vi "StateDrivebase.vi"(0 "Master State In":T1(ring)) -> ()   [LabVIEW 2020]
doc: "This VI performs all of the calculations and decisions related to the swerve drive."
uses:
  GlobalDriverStationCommands.vi
  GlobalDriverStationData.vi
  GlobalPoseAndTargeting.vi
  GlobalDrivebase.vi
panel:
  in  "Max Strafing While Balancing":dbl=0.25
  in  "Speed Cap Decceleration Limit (/s)":dbl=20.0
  in  "PID Tuning Anti-Drift":T2={"Kp"=0.00045, "Ki"=0.0, "Kd"=0.0, "N-Diff"=3, "N-Int"=10, "Int Error Window"=90.0, "Max Ouput"=1.0, "Min Output"=-1.0, "Square Derivative"=FALSE, "N-Prop"=5} {"N-Prop" min=1; "Int Error Window" min=0.0; "N-Int" min=2; "N-Diff" min=2; "Kd" min=0.0; "Ki" min=0.0; "Kp" min=0.0}
  in  "Anti-Drift Deceleration Hysteresis (ms)":u32=1
  out "Anti-Drift Control":bool
  in  "Anti-Drift Strafe Deadband (ft/s)":dbl=3.0
  in  "Manually Disable Anti-Drift":bool
  in  "PID Tuning Heading Lock":T3={"Kp"=0.0045, "Ki"=0.01, "Kd"=0.0002, "N-Diff"=10, "N-Int"=10, "Int Error Window"=30.0, "Max Ouput"=1.0, "Min Output"=-1.0} {"Int Error Window" min=0.0; "N-Int" min=2; "N-Diff" min=2; "Kd" min=0.0; "Ki" min=0.0; "Kp" min=0.0}
  out "PID Plots":T4(graph)
  in  "Manual Fudge Factor Heading Lock (deg)":dbl=10.0
  in  "Plot PID":bool
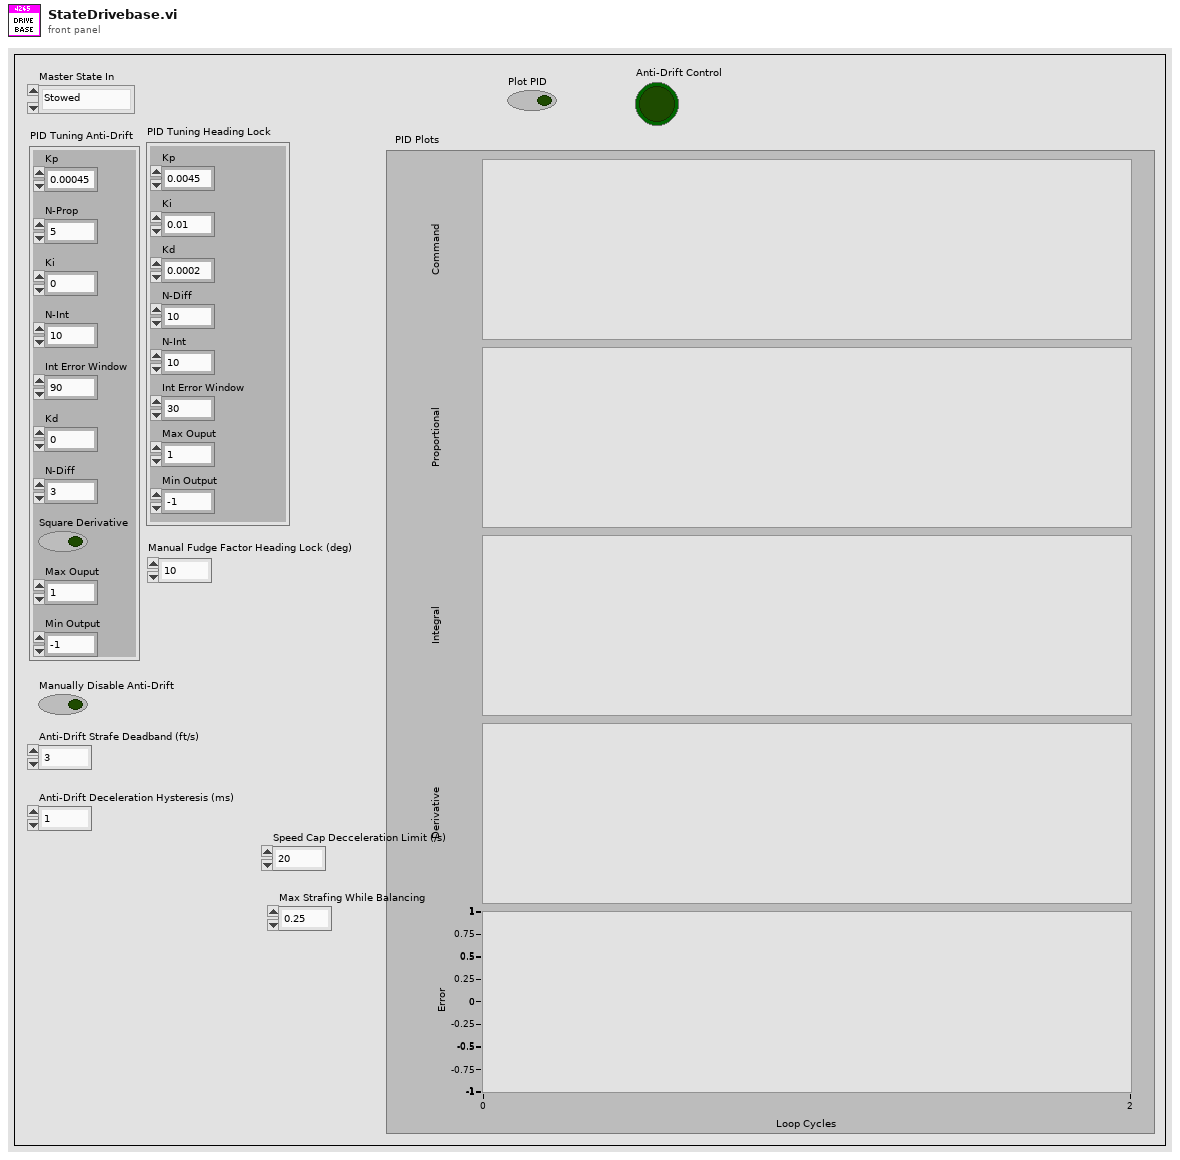
[diagram p1: front panel]
types:
  T1 = enum16{"Stowed", "Balancing", "Scoring", "Hoppering", "Ground", "Shelf"}
  T2 = cluster{"Kp":dbl, "Ki":dbl, "Kd":dbl, "N-Diff":i32, "N-Int":i32, "Int Error Window":dbl, "Max Ouput":dbl, "Min Output":dbl, "Square Derivative":bool, "N-Prop":i32}
  T3 = cluster{"Kp":dbl, "Ki":dbl, "Kd":dbl, "N-Diff":i32, "N-Int":i32, "Int Error Window":dbl, "Max Ouput":dbl, "Min Output":dbl}
  T4 = cluster{"Command":dbl, "Proportional":dbl, "Integral":dbl, "Derivative":dbl, "Goal":dbl}
  T5 = cluster{"Current Setpoints[0]":dbl, "Current Setpoints[1]":dbl, "Current Setpoints[2]":dbl, "Current Setpoints[3]":dbl, "Current Setpoints[4]":dbl, "Current Setpoints[5]":dbl, "Current Setpoints[6]":dbl, "Current Setpoints[7]":dbl, "Current Setpoints[8]":dbl}
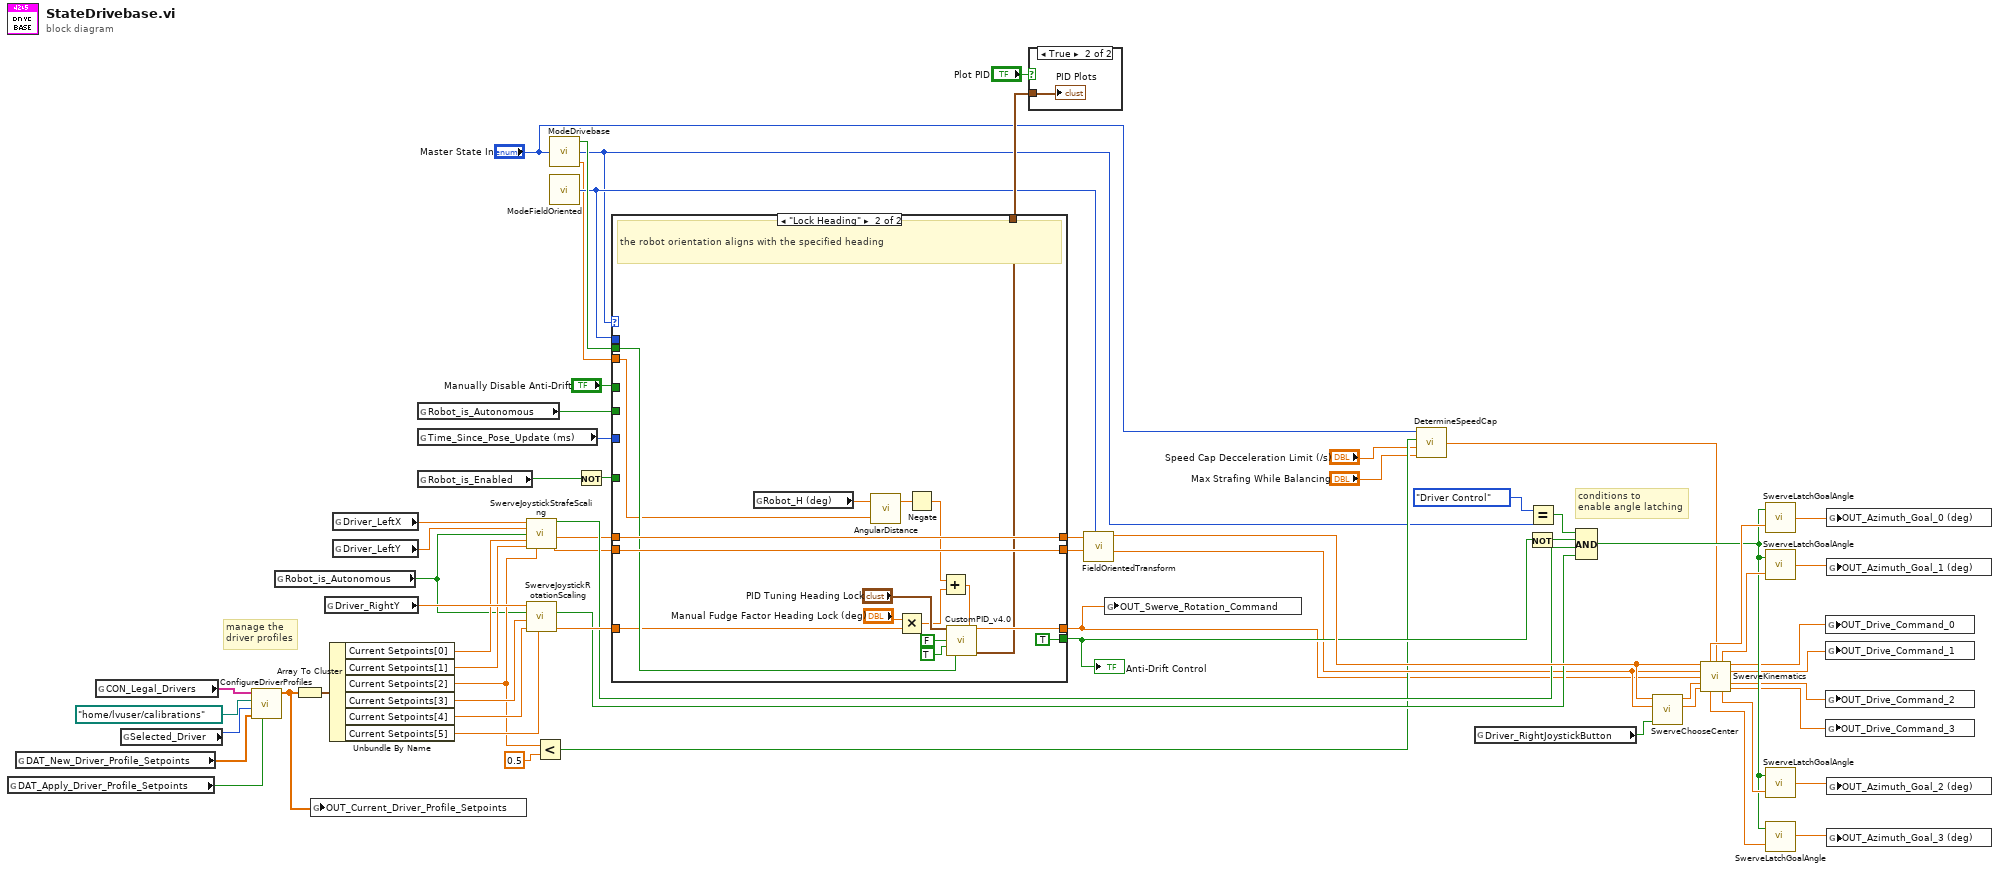
[diagram p0: block diagram]
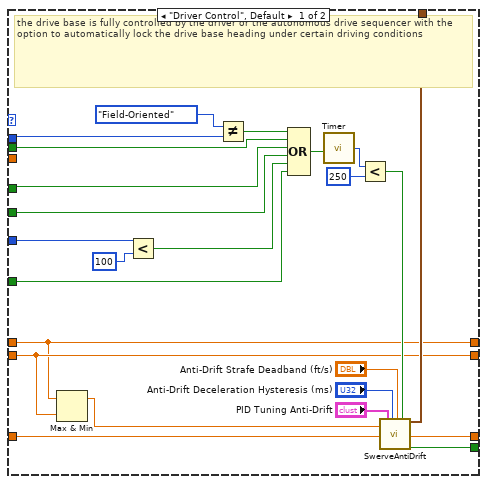
[diagram p3: hidden frame]
diagram:
  # "conditions to\nenable angle latching"
  # "manage the\ndriver profiles"
  n1 = global read "GlobalDrivebase.vi" "DAT_Apply_Driver_Profile_Setpoints"() -> (w20:bool)
  n2 = global read "GlobalDrivebase.vi" "DAT_New_Driver_Profile_Setpoints"() -> (w21:dbl[])
  n3 = global read "GlobalDrivebase.vi" "CON_Legal_Drivers"() -> (w19:string[])
  n4 = global read "GlobalDriverStationData.vi" "Selected_Driver"() -> (w31:i32)
  n5 = call "ConfigureDriverProfiles.vi"("Apply New Setpoint"=w20, "New Setpoints"=w21, "Selected Driver"=w31, "Setpoint Save Location"=path "/home/lvuser/calibrations", "Driver Profile Names"=w19) -> ("Current Setpoints"=w9:dbl[])  [unwired: 6 in]
  n6 = global read "GlobalDriverStationData.vi" "Robot_is_Autonomous"() -> (w27:bool)
  n7 = Array To Cluster(array=w9) -> (cluster=w30:T5)
  n8 = global write "GlobalDrivebase.vi" "OUT_Current_Driver_Profile_Setpoints"(w9) -> ()
  n9 = global read "GlobalDriverStationCommands.vi" "Driver_RightY"() -> (w49:dbl)
  n10 = Unbundle By Name(w30) -> ("Current Setpoints[0]"=w39:dbl, "Current Setpoints[1]"=w38:dbl, "Current Setpoints[2]"=w28:dbl, "Current Setpoints[3]"=w37:dbl, "Current Setpoints[4]"=w36:dbl, "Current Setpoints[5]"=w35:dbl)
  n11 = global read "GlobalDriverStationCommands.vi" "Driver_LeftX"() -> (w52:dbl)
  n12 = global read "GlobalDriverStationCommands.vi" "Driver_LeftY"() -> (w51:dbl)
  n13 = global read "GlobalDriverStationData.vi" "Robot_is_Autonomous"() -> (w57:bool)
  n14 = global read "GlobalPoseAndTargeting.vi" "Time_Since_Pose_Update (ms)"() -> (w58:u32)
  n15 = global read "GlobalDriverStationData.vi" "Robot_is_Enabled"() -> (w6:bool)
  n16 = call "SwerveJoystickStrafeScaling.vi"("Raw Joystick X"=w52, "Raw Joystick Y"=w51, "Auto Control"=w27, "Strafe Deadband"=w39, "Strafe Scaling"=w38, "Strafe Maximum"=w28) -> ("In Deadband"=w45:bool, "Scaled Joystick X"=w25:dbl, "Scaled Joystick Y"=w26:dbl)  [unwired: 7 in]
  n17 = call "SwerveJoystickRotationScaling.vi"("Rotation Maximum"=w35, "Rotation Scaling"=w36, "Rotation Deadband"=w37, "Auto Control"=w27, "Raw Joystick Rotation"=w49) -> ("Scaled Joystick Rotation"=w50:dbl, "In Deadband"=w46:bool)  [unwired: 4 in]
  n18 = Less?(x=w28, y=0.5) -> (x < y?=w22:bool)
  n19 = call "ModeDrivebase.vi"("Master State In"="Master State In") -> ("Drive Mode Change"=w55:bool, "Drive Mode"=w4:enum16{"Driver Control", "Lock Heading"}, "Locked Heading (deg)"=w7:dbl)
  n20 = call "ModeFieldOriented.vi"() -> ("Orientation Mode"=w41:enum16{"Robot-Oriented", "Field-Oriented"})  [unwired: 1 in]
  n21 = Not(x=w6) -> (.not. x?=w5:bool)
  n22 = case shown="\"Lock Heading\"" w4 {
    tunnel: [w68 w104] -> w40
    tunnel: [w67 w102] -> w64
    tunnel: w25 -> [w67 w102]
    tunnel: w26 -> [w68 w104]
    tunnel: w50 -> [w79 w90]
    tunnel: [w80 w101] -> w18
    tunnel: [w85 TRUE ("auto rot control")] -> w47
    tunnel: w41 -> [w86 _]
    tunnel: w57 -> [w83 _]
    tunnel: w55 -> [w77 w97]
    tunnel: w58 -> [w88 _]
    tunnel: [w82 w96] -> w56
    tunnel: "Manually Disable Anti-Drift" -> [w81 _]
    tunnel: w5 -> [w71 _]
    tunnel: w7 -> [_ w91]
    frame "Driver Control", Default {
      # "the drive base is fully controlled by the driver or the autonomous drive sequencer with the option to automatically lock the drive base heading under certain driving conditions"
      n23 = Max & Min(x=w67, y=w68) -> (max(x,y)=w66:dbl)  [unwired: 1 out]
      n24 = Less?(x=w88, y=u32 100) -> (x < y?=w84:bool)
      n25 = Not Equal?(x=enum16{"Robot-Oriented", "Field-Oriented"}."Field-Oriented", y=w86) -> (x != y?=w76:bool)
      n26 = Compound Arithmetic op=OR(w76, w77, w81, w83, w84, w71) -> (w74:bool)
      n27 = call "Timer.vi"("Reset Timer"=w74) -> ("Time (ms)"=w75:u32)
      n28 = Less?(x=w75, y=u32 250) -> (x < y?=w72:bool)
      n29 = call "SwerveAntiDrift.vi"("Max Driver Translation Joystick"=w66, "Driver Rotation Joystick"=w79, "PID Tuning Parameters"="PID Tuning Anti-Drift", "Deceleration Hysteresis (ms)"="Anti-Drift Deceleration Hysteresis (ms)", "Strafe Deadband (ft/s)"="Anti-Drift Strafe Deadband (ft/s)", "External Disables"=w72) -> ("Controller Summary"=w82:T4, "Joystick Rotation"=w80:dbl, "Anti-Drift"=w85:bool)  [unwired: 11 in]
    }
    frame "Lock Heading" {
      # "the robot orientation aligns with the specified heading"
      n30 = global read "GlobalPoseAndTargeting.vi" "Robot_H (deg)"() -> (w105:dbl)
      n31 = call "AngularDistance.vi"("Goal Angle (deg) [0,360]"=w91, "Current Angle (deg) [-Inf,+Inf]"=w105) -> ("Signed Angular Distance (deg) [-180,+180]"=w95:dbl)  [unwired: 1 out]
      n32 = Multiply(x="Manual Fudge Factor Heading Lock (deg)", y=w90) -> (x*y=w94:dbl)
      n33 = Negate(x=w95) -> (-x=w93:dbl)
      n34 = Add(x=w93, y=w94) -> (x+y=w92:dbl)
      n35 = call "CustomPID_v4.0.vi"("PID Tuning Parameters"="PID Tuning Heading Lock", "Custom Error Calculation"=w92, "Reset on Goal Change ?"=FALSE, "Use Custom Error Calculation ?"=TRUE, "Reinit"=w97) -> ("Command"=w101:dbl, "Controller Summary"=w96:T4)  [unwired: 7 in, 2 out]
    }
  }
  "Anti-Drift Control" <- w47
  n36 = case shown="True" "Plot PID" {
    tunnel: w56 -> [_ w106]
    frame False {
    }
    frame True {
      "PID Plots" <- w106
    }
  }
  n37 = call "FieldOrientedTransform.vi"("Orientation Mode"=w41, "Joystick Y"=w40, "Joystick X"=w64) -> ("Joystick Y'"=w42:dbl, "Joystick X'"=w48:dbl)  [unwired: 7 in]
  n38 = global write "GlobalDrivebase.vi" "OUT_Swerve_Rotation_Command"(w18) -> ()
  n39 = call "DetermineSpeedCap.vi"("Max Strafing While Balancing"="Max Strafing While Balancing", "Speed Cap Decceleration Limit (/s)"="Speed Cap Decceleration Limit (/s)", "Driver Profile Doesn't Want to Shift"=w22, "Master State"="Master State In") -> ("Speed Cap [0,1]"=w23:dbl)
  n40 = global read "GlobalDriverStationCommands.vi" "Driver_RightJoystickButton"() -> (w54:bool)
  n41 = Not(x=w47) -> (.not. x?=w44:bool)
  n42 = Equal?(x=enum16{"Driver Control", "Lock Heading"}."Driver Control" ("Drive Mode"), y=w4) -> (x = y?=w43:bool)
  n43 = Compound Arithmetic op=AND(w43, w44, w45, w46) -> (w24:bool)
  n44 = call "SwerveChooseCenter.vi"("Defensive Driving Trigger"=w54, "Joystick Y"=w42, "Joystick X"=w48) -> ("Cy (in)"=w33:dbl, "Cx (in)"=w34:dbl)  [unwired: 5 in]
  n45 = call "SwerveKinematics.vi"("Joystick X"=w48, "Saturation Velocity (ul)"=w23, "Joystick Y"=w42, "Joystick Rotation"=w18, "Cx (in)"=w34, "Cy (in)"=w33) -> ("Module 0 Angle (deg)"=w63:dbl, "Module 1 Angle (deg)"=w62:dbl, "Module 0 Velocity Command (ul)"=w13:dbl, "Module 1 Velocity Command (ul)"=w12:dbl, "Module 2 Velocity Command (ul)"=w11:dbl, "Module 3 Angle (deg)"=w59:dbl, "Module 2 Angle (deg)"=w60:dbl, "Module 3 Velocity Command (ul)"=w10:dbl)  [unwired: 2 in]
  n46 = call "SwerveLatchGoalAngle.vi"("Raw Goal Angle"=w63, "In Deadband"=w24) -> ("Latched Goal Angle"=w17:dbl)
  n47 = call "SwerveLatchGoalAngle.vi"("Raw Goal Angle"=w62, "In Deadband"=w24) -> ("Latched Goal Angle"=w16:dbl)
  n48 = call "SwerveLatchGoalAngle.vi"("Raw Goal Angle"=w60, "In Deadband"=w24) -> ("Latched Goal Angle"=w15:dbl)
  n49 = call "SwerveLatchGoalAngle.vi"("Raw Goal Angle"=w59, "In Deadband"=w24) -> ("Latched Goal Angle"=w14:dbl)
  n50 = global write "GlobalDrivebase.vi" "OUT_Drive_Command_0"(w13) -> ()
  n51 = global write "GlobalDrivebase.vi" "OUT_Drive_Command_1"(w12) -> ()
  n52 = global write "GlobalDrivebase.vi" "OUT_Drive_Command_2"(w11) -> ()
  n53 = global write "GlobalDrivebase.vi" "OUT_Drive_Command_3"(w10) -> ()
  n54 = global write "GlobalDrivebase.vi" "OUT_Azimuth_Goal_0 (deg)"(w17) -> ()
  n55 = global write "GlobalDrivebase.vi" "OUT_Azimuth_Goal_1 (deg)"(w16) -> ()
  n56 = global write "GlobalDrivebase.vi" "OUT_Azimuth_Goal_2 (deg)"(w15) -> ()
  n57 = global write "GlobalDrivebase.vi" "OUT_Azimuth_Goal_3 (deg)"(w14) -> ()
